vi "Main3Diposits.vi"() -> ()   [LabVIEW 2019]
panel:
  out "OPERACIÓ NORMAL":bool
  out "ALARMA":bool
  in  "stop":bool
  out "Boolean 3":bool
  out "Boolean 2":bool
  out "Boolean":bool
  in  "Límit buit":dbl(slide) scale=0.0..10000.0
  in  "Dipòsit 3":dbl(slide) scale=0.0..10000.0
  in  "Dipòsit 2":dbl(slide) scale=0.0..10000.0
  in  "Dipòsit 1":dbl(slide) scale=0.0..10000.0
  # "DISSENY D'UN CIRCUIT LÒGIC PER A UNA PLANTA DEPURADORA"
  # "ESTAT PLANTA\nDEPURADORA"
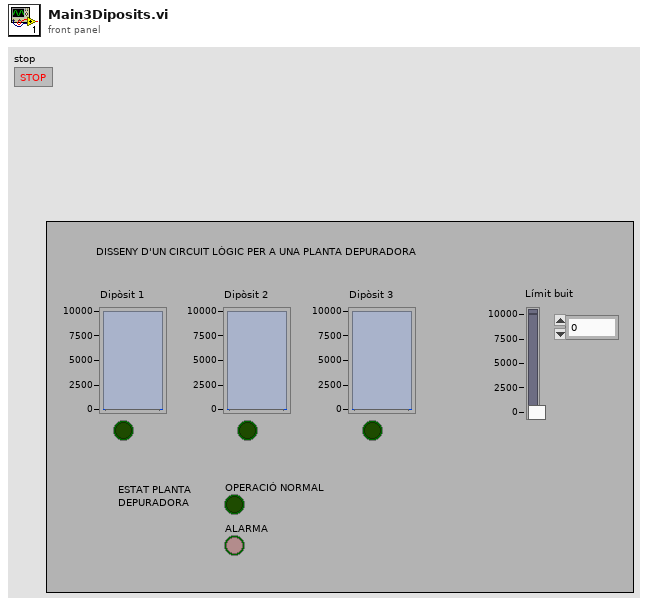
[diagram p1: front panel]
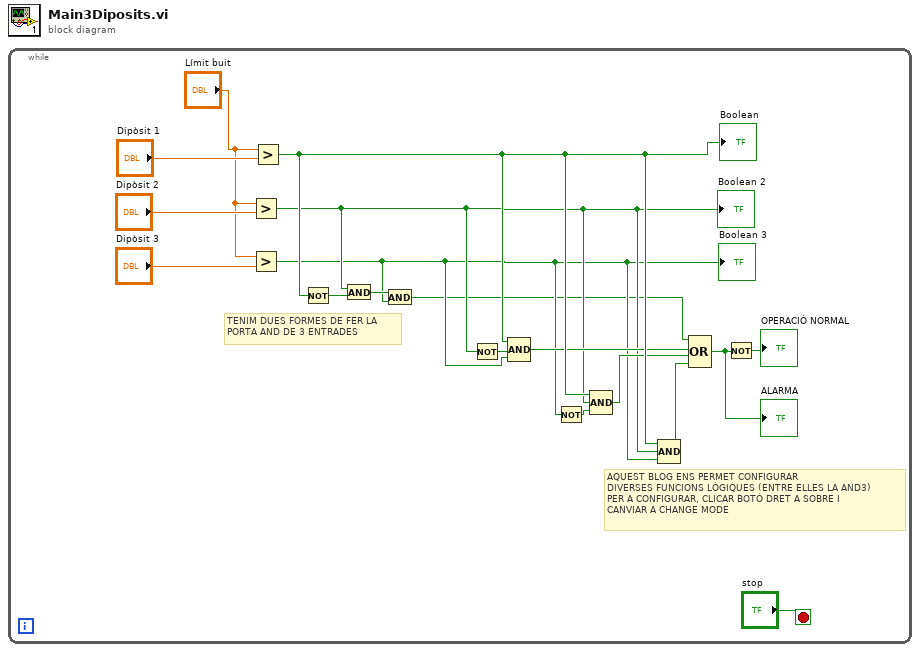
[diagram p0: block diagram]
diagram:
  n1 = while {
    stop <- "stop" stop-if-true
    # "AQUEST BLOG ENS PERMET CONFIGURAR\nDIVERSES FUNCIONS LÒGIQUES (ENTRE ELLES LA AND3)\nPER A CONFIGURAR, CLICAR BOTÓ DRET A SOBRE I \nCANVIAR A CHANGE MODE"
    # "TENIM DUES FORMES DE FER LA \nPORTA AND DE 3 ENTRADES"
    n2 = Greater?(x="Límit buit", y="Dipòsit 2") -> (0:w4:bool)
    "Boolean 2" <- w4
    n3 = Greater?(x="Límit buit", y="Dipòsit 3") -> (0:w2:bool)
    "Boolean 3" <- w2
    n4 = Greater?(x="Límit buit", y="Dipòsit 1") -> (0:w11:bool)
    "Boolean" <- w11
    n5 = Not(x=w11) -> (.not. x?=w5:bool)
    n6 = And(x=w4, y=w5) -> (x .and. y?=w3:bool)
    n7 = And(x=w3, y=w2) -> (x .and. y?=w1:bool)
    n8 = Not(x=w4) -> (.not. x?=w13:bool)
    n9 = Compound Arithmetic op=AND(w11, w13, w2) -> (w8:bool)
    n10 = Not(x=w2) -> (.not. x?=w12:bool)
    n11 = Compound Arithmetic op=AND(w11, w4, w12) -> (w9:bool)
    n12 = Compound Arithmetic op=AND(w11, w4, w2) -> (w10:bool)
    n13 = Compound Arithmetic op=OR(w1, w8, w9, w10) -> (w6:bool)
    "ALARMA" <- w6
    n14 = Not(x=w6) -> (.not. x?=→"OPERACIÓ NORMAL":bool)
  }
